vi "DHE_DRV_get_guide_mode.vi"(11 "error in (no error)":errorcluster) -> (6 "guide_mode":bool, 15 "error out":errorcluster)   [LabVIEW 2016]
doc: "This VI closes the I/O interface with the instrument."
uses:
  c/lib/libarcDHE.so
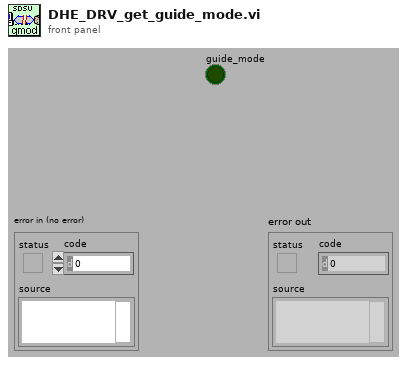
[diagram p1: front panel]
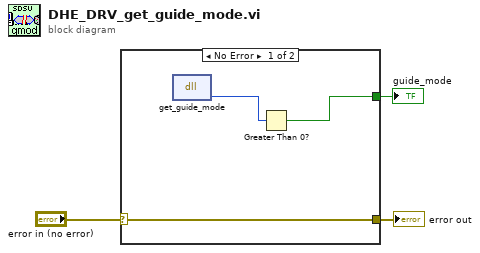
[diagram p0: block diagram]
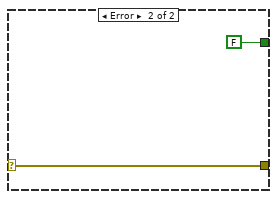
[diagram p2: hidden frame]
diagram:
  n1 = case shown="No Error" "error in (no error)" {
    selector: "error in (no error)" -> [w6 w8]
    tunnel: [w4 FALSE] -> w1
    tunnel: [w6 w8] -> w3
    frame No Error {
      n2 = dll-call lib="home/simager/panview/PAN/Modules/SDSU/private/c/lib/libarcDHE.so" fn="get_guide_mode" label="get_expdelay"() -> ("return type"=w5:i32)  [unwired: 3 in, 2 out]
      n3 = Greater Than 0?(x=w5) -> (x > 0?=w4:bool)
    }
    frame Error {
    }
  }
  "error out" <- w3
  "guide_mode" <- w1
